vi "m1m3_getSample_ForceActuatorStatus.vi"(8 "error in (no error)":errorcluster, 11 "ForceActuatorStatus_Ctl":T1) -> (0 "error out":errorcluster, 2 "function return":i32, 3 "ForceActuatorStatus_Ctl out":T1)   [LabVIEW 2016, in "SALLV_m1m3.lvlib"]
doc: "int m1m3_shm_getSample_ForceActuatorStatusLV(m1m3_ForceActuatorStatusLV *ForceActuatorStatus_Ctl );"
uses:
  SALLV_m1m3.lvlib
  DataTypes/ForceActuatorStatus.ctl
  SALLV_m1m3.so
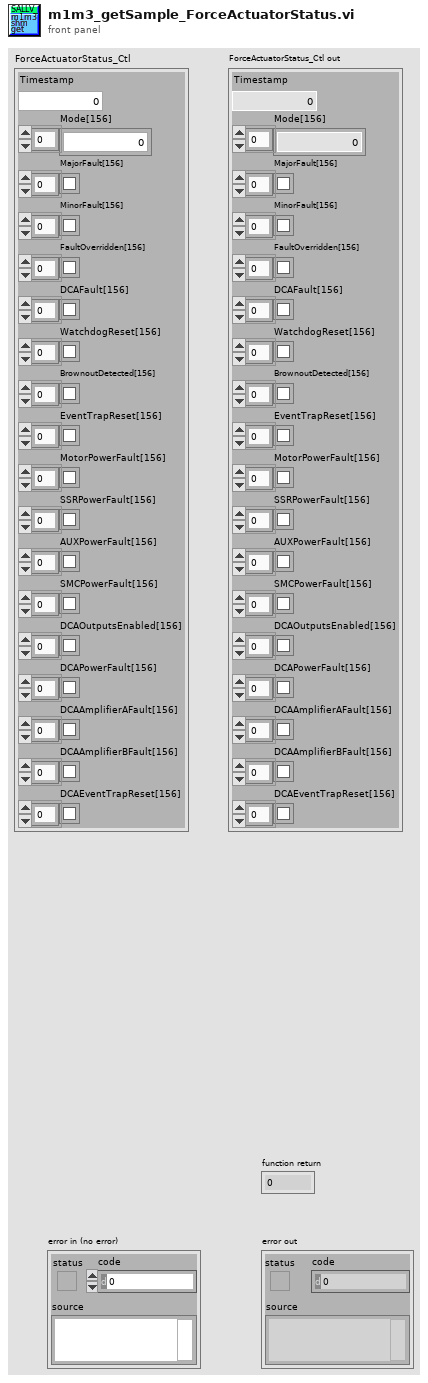
[diagram p1: front panel]
types:
  T1 = typedef "SALLV_m1m3.lvlib/ForceActuatorStatus.ctl" = cluster{"Timestamp":dbl, "Mode[156]":u8[], "MajorFault[156]":bool[], "MinorFault[156]":bool[], "FaultOverridden[156]":bool[], "DCAFault[156]":bool[], "WatchdogReset[156]":bool[], "BrownoutDetected[156]":bool[], "EventTrapReset[156]":bool[], "MotorPowerFault[156]":bool[], "SSRPowerFault[156]":bool[], "AUXPowerFault[156]":bool[], "SMCPowerFault[156]":bool[], "DCAOutputsEnabled[156]":bool[], "DCAPowerFault[156]":bool[], "DCAAmplifierAFault[156]":bool[], "DCAAmplifierBFault[156]":bool[], "DCAEventTrapReset[156]":bool[]}
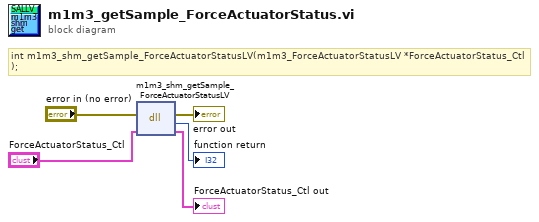
[diagram p0: block diagram]
diagram:
  # "int m1m3_shm_getSample_ForceActuatorStatusLV(m1m3_ForceActuatorStatusLV *ForceActuatorStatus_Ctl );"
  n1 = dll-call lib="opt/CODE/ts_m1m3supporteui/SALLV_m1m3/SALLV_m1m3.*" fn="m1m3_shm_getSample_ForceActuatorStatusLV"(error in="error in (no error)", "ForceActuatorStatus_Ctl"="ForceActuatorStatus_Ctl") -> (error out=→"error out":errorcluster, →"function return":i32, "ForceActuatorStatus_Ctl"=→"ForceActuatorStatus_Ctl out":T1)  [unwired: 2 in, 1 out]
